vi "q3 decimal to binary.vi"() -> ()   [LabVIEW 2025]
panel:
  out "binary":dbl
  in  "decimal":dbl
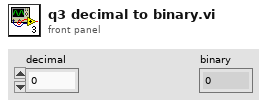
[diagram p1: front panel]
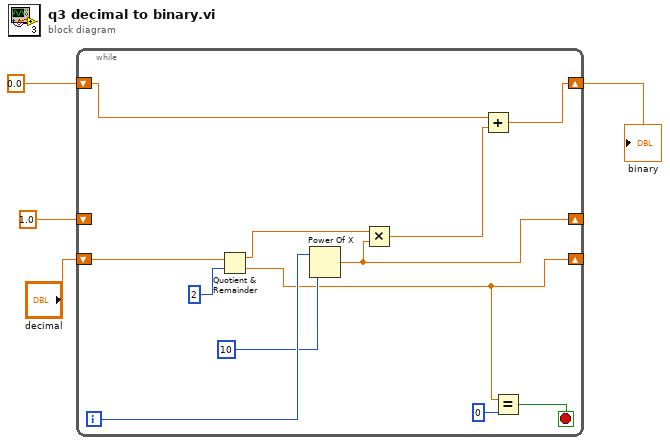
[diagram p0: block diagram]
diagram:
  n1 = while {
    shift-right: [w9] -> w1
    shift-left: 0.0 -> [w15]
    shift-right: [w8] -> _
    shift-left: 1.0 -> [_]
    shift-right: [w7] -> _
    shift-left: "decimal" -> [w12]
    i -> [w14]
    stop <- w11 stop-if-true
    n2 = Quotient & Remainder(x=w12, y=2) -> (x-y*floor(x/y)=w5:dbl, floor(x/y)=w7:dbl)
    n3 = Power Of X(1:10, 2:w14) -> (0:w8:dbl)
    n4 = Multiply(x=w5, y=w8) -> (x*y=w6:dbl)
    n5 = Add(x=w15, y=w6) -> (x+y=w9:dbl)
    n6 = Equal?(x=w7, y=0) -> (x = y?=w11:bool)
  }
  "binary" <- w1
